vi "SetPackBaudrate.vi"(0 "handle in":i32, 1 "UnitAddress(0)":u16, 5 "error in":errorcluster, 7 "BaudRate (19200)":enum32{"9600", "19200", "38400", "57600"}(ring)=enum."19200", 9 "Delay(6)":u16=6) -> (14 "handle out":i32, 19 "error out":errorcluster)   [LabVIEW 2014, in "Sixpack - Driver.lvlib"]
uses:
  Sixpack - Driver.lvlib
  DLL/PackDLL.dll
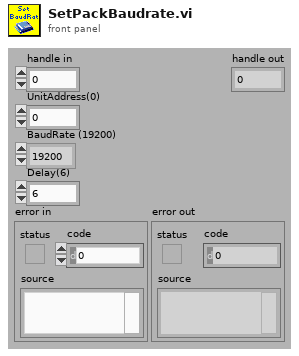
[diagram p1: front panel]
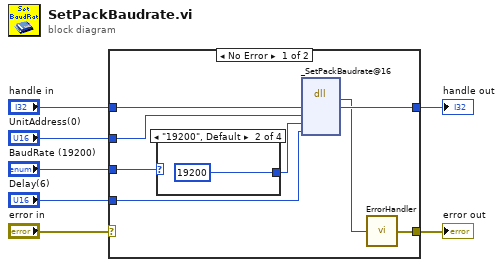
[diagram p0: block diagram]
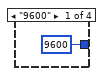
[diagram p2: hidden frame]
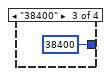
[diagram p3: hidden frame]
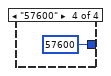
[diagram p4: hidden frame]
diagram:
  n1 = case shown="No Error" "error in" {
    selector: "error in" -> [_ w20]
    tunnel: "UnitAddress(0)" -> [w15 _]
    tunnel: "handle in" -> [w14 w21]
    tunnel: "Delay(6)" -> [w13 _]
    tunnel: [w12 w21] -> w4
    tunnel: "BaudRate (19200)" -> [w11 _]
    tunnel: [w8 w20] -> w2
    frame No Error {
      n2 = case shown="\"19200\", Default" w11 {
        tunnel: [9600 ("BaudRate") 19200 ("BaudRate") 38400 ("BaudRate") 57600 ("BaudRate")] -> w10
        frame "9600" {
        }
        frame "19200", Default {
        }
        frame "38400" {
        }
        frame "57600" {
        }
      }
      n3 = dll-call lib="D:/CS-Source/LV2014/GPL/instr.lib/SixPack/PackDLL/DLL/PackDLL.dll" fn="_SetPackBaudrate@16" label="SetPackBaudrate"("handle"=w14, "UnitAddress"=w15, "BaudRate"=w10, "Delay"=w13) -> ("BOOLEAN"=w9:i8, "handle"=w12:i32)  [unwired: 6 in, 2 out]
      n4 = call "ErrorHandler.vi"("BOOLEAN"=w9) -> ("error out"=w8:errorcluster)
    }
    frame Error {
    }
  }
  "handle out" <- w4
  "error out" <- w2
